vi "Identity Matrix.vi"(11 "Size of Square Matrix":i32=1000) -> (3 "Identity Matrix":T1)   [LabVIEW 2019]
uses:
  <vilib>/silver_ctls/ArrayMatrixCluster/Real Matrix NI_Silver.ctl
  <vilib>/Analysis/Matrix/Datatypes/RealMatrix.ctl
  <vilib>/Analysis/Matrix/NI_Matrix.lvlib
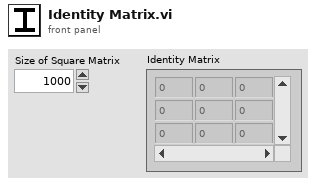
[diagram p1: front panel]
types:
  T1 = typedef "Real Matrix NI_Silver.ctl" = dbl[][]
  T2 = typedef "NI_Matrix.lvlib/RealMatrix.ctl" = dbl[][]
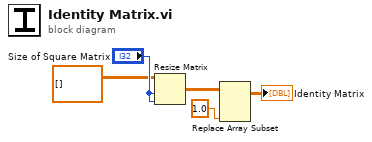
[diagram p0: block diagram]
diagram:
  n1 = Resize Matrix(1:"Size of Square Matrix", 2:"Size of Square Matrix", 4:T2 [] ("matrix")) -> (0:w4:T2)
  n2 = Replace Array Subset(array=w4, new element=1.0 ("new diagonal/fill element")) -> (→"Identity Matrix":T2)  [unwired: 2 in]
